vi "QueryParameters.vi"(8 "error in (no error)":errorcluster, 11 "HRS_Spectrometer in":refnum<class "HRS_Spectrometer.lvclass">) -> (0 "error out":errorcluster, 3 "HRS_Spectrometer out":refnum<class "HRS_Spectrometer.lvclass">)   [LabVIEW 2023, in "Spectrometer Library.lvlib" / "HRS_Spectrometer.lvlib" / "HRS_Spectrometer.lvclass"]
uses:
  HRS_Spectrometer.lvclass
  HRS_Spectrometer.lvclass/HRS_Spectrometer.ctl
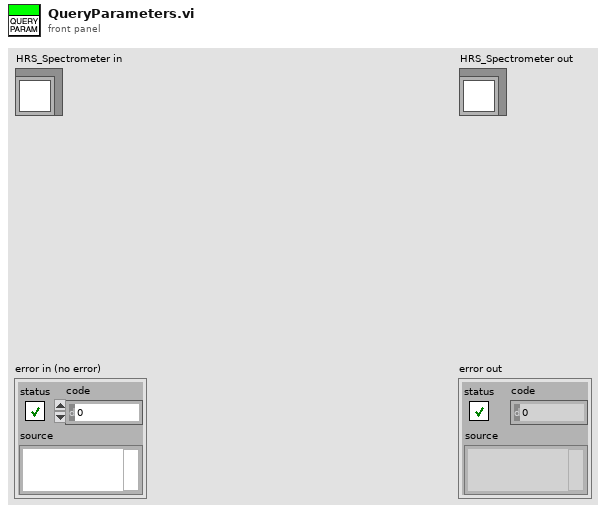
[diagram p1: front panel]
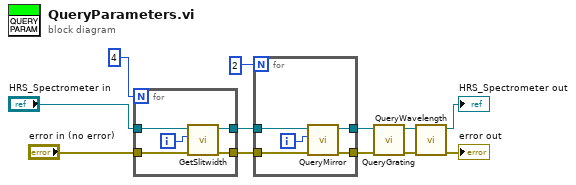
[diagram p0: block diagram]
diagram:
  n1 = for {
    N: 4 -> [_]
    tunnel: "HRS_Spectrometer in" -> [w16]
    tunnel: [w15] -> w9
    tunnel: [w14] -> w12
    tunnel: "error in (no error)" -> [w13]
    i -> [w17]
    n2 = call-dynamic "GetSlitwidth.vi"("error in (no error)"=w13, "Slit"=w17, "HRS_Spectrometer in"=w16) -> ("error out"=w14:errorcluster, "HRS_Spectrometer out"=w15:refnum<class "HRS_Spectrometer.lvclass">)  [unwired: 7 in]
  }
  n3 = for {
    N: 2 -> [_]
    tunnel: w9 -> [w21]
    tunnel: [w20] -> w8
    tunnel: [w19] -> w11
    tunnel: w12 -> [w18]
    i -> [w22]
    n4 = call-dynamic "QueryMirror.vi"("error in (no error)"=w18, "Mirror"=w22, "HRS_Spectrometer in"=w21) -> ("error out"=w19:errorcluster, "HRS_Spectrometer out"=w20:refnum<class "HRS_Spectrometer.lvclass">)  [unwired: 7 in]
  }
  n5 = call-dynamic "QueryGrating.vi"("error in (no error)"=w11, "HRS_Spectrometer in"=w8) -> ("error out"=w10:errorcluster, "HRS_Spectrometer out"=w7:refnum<class "HRS_Spectrometer.lvclass">)  [unwired: 8 in]
  n6 = call-dynamic "QueryWavelength.vi"("error in (no error)"=w10, "HRS_Spectrometer in"=w7) -> ("error out"=→"error out":errorcluster, "HRS_Spectrometer out"=→"HRS_Spectrometer out":refnum<class "HRS_Spectrometer.lvclass">)  [unwired: 8 in]
